vi "Drive and Climb Logging.vi"   [LabVIEW 2016]
uses:
  Robot Global Data.vi
  Drive and Climb Logging Values.vi
types:
  T1 = typedef "WPI_DriverStationRobotMode2.ctl" = enum16{"Autonomous Disabled", "Autonomous Enabled", "Teleop Disabled", "Teleop Enabled", "Disconnected", "Finish", "Test Disabled", "Test Enabled", "Emergency Stopped"}
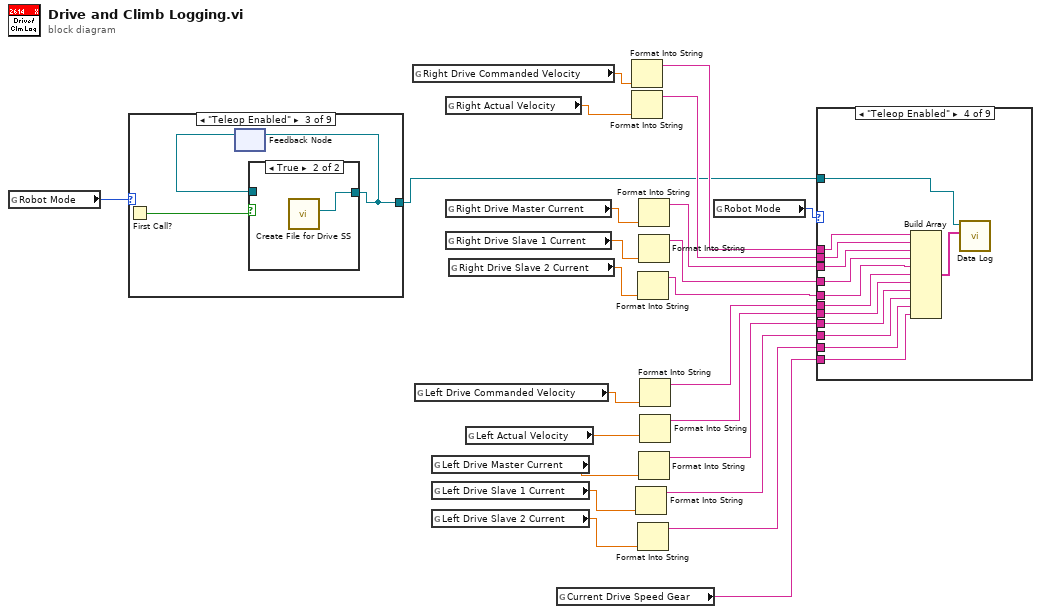
[diagram p0: block diagram]
diagram:
  n1 = global read "Robot Global Data.vi" "Robot Mode"() -> (w19:T1)
  n2 = case shown="\"Teleop Enabled\"" w19 {
    tunnel: [_ _ w25 _ _ _ _ _ _] -> w18
    frame "Autonomous Enabled" {
    }
    frame "Teleop Disabled", Default {
    }
    frame "Teleop Enabled" {
      n3 = First Call?() -> (First Call?: T/F=w27:bool)
      n4 = feedback #1() -> (w26:refnum<file>)  [unwired: 1 in]
      n5 = case shown="True" w27 {
        tunnel: [w28 w29] -> w25
        tunnel: w26 -> [w28 _]
        frame False {
        }
        frame True {
          n6 = call "Create File for Drive SS.vi"() -> ("File Reference Out"=w29:refnum<file>)  [unwired: 11 in]
        }
      }
      n7 = feedback-in #1(w25) -> ()
    }
    frame "Disconnected" {
    }
    frame "Finish" {
    }
    frame "Test Disabled" {
    }
    frame "Test Enabled" {
    }
    frame "Emergency Stopped" {
    }
    frame "Autonomous Disabled" {
    }
  }
  n8 = global read "Drive and Climb Logging Values.vi" "Right Drive Commanded Velocity"() -> (w13:dbl)
  n9 = global read "Drive and Climb Logging Values.vi" "Left Drive Commanded Velocity"() -> (w14:dbl)
  n10 = global read "Drive and Climb Logging Values.vi" "Left Drive Master Current"() -> (w12:dbl)
  n11 = global read "Drive and Climb Logging Values.vi" "Left Drive Slave 1 Current"() -> (w11:dbl)
  n12 = global read "Drive and Climb Logging Values.vi" "Left Drive Slave 2 Current"() -> (w10:dbl)
  n13 = global read "Drive and Climb Logging Values.vi" "Right Actual Velocity"() -> (w17:dbl)
  n14 = global read "Drive and Climb Logging Values.vi" "Right Drive Master Current"() -> (w6:dbl)
  n15 = global read "Drive and Climb Logging Values.vi" "Right Drive Slave 1 Current"() -> (w5:dbl)
  n16 = global read "Drive and Climb Logging Values.vi" "Right Drive Slave 2 Current"() -> (w4:dbl)
  n17 = global read "Drive and Climb Logging Values.vi" "Left Actual Velocity"() -> (w15:dbl)
  n18 = global read "Drive and Climb Logging Values.vi" "Current Drive Speed Gear"() -> (w16:string)
  n19 = Format Into String(w13) -> (resulting string=w24:string)  [unwired: 3 in, 1 out]
  n20 = Format Into String(w17) -> (resulting string=w23:string)  [unwired: 3 in, 1 out]
  n21 = Format Into String(w11) -> (resulting string=w8:string)  [unwired: 3 in, 1 out]
  n22 = Format Into String(w4) -> (resulting string=w1:string)  [unwired: 3 in, 1 out]
  n23 = Format Into String(w10) -> (resulting string=w7:string)  [unwired: 3 in, 1 out]
  n24 = Format Into String(w6) -> (resulting string=w3:string)  [unwired: 3 in, 1 out]
  n25 = Format Into String(w5) -> (resulting string=w2:string)  [unwired: 3 in, 1 out]
  n26 = Format Into String(w12) -> (resulting string=w9:string)  [unwired: 3 in, 1 out]
  n27 = Format Into String(w14) -> (resulting string=w22:string)  [unwired: 3 in, 1 out]
  n28 = Format Into String(w15) -> (resulting string=w21:string)  [unwired: 3 in, 1 out]
  n29 = global read "Robot Global Data.vi" "Robot Mode"() -> (w20:T1)
  n30 = case shown="\"Teleop Enabled\"" w20 {
    tunnel: w24 -> [_ _ _ w41 _ _ _ _ _]
    tunnel: w23 -> [_ _ _ w40 _ _ _ _ _]
    tunnel: w22 -> [_ _ _ w39 _ _ _ _ _]
    tunnel: w21 -> [_ _ _ w33 _ _ _ _ _]
    tunnel: w16 -> [_ _ _ w38 _ _ _ _ _]
    tunnel: w18 -> [_ _ _ w37 _ _ _ _ _]
    tunnel: w9 -> [_ _ _ w36 _ _ _ _ _]
    tunnel: w8 -> [_ _ _ w35 _ _ _ _ _]
    tunnel: w7 -> [_ _ _ w34 _ _ _ _ _]
    tunnel: w3 -> [_ _ _ w32 _ _ _ _ _]
    tunnel: w2 -> [_ _ _ w31 _ _ _ _ _]
    tunnel: w1 -> [_ _ _ w30 _ _ _ _ _]
    frame "Autonomous Disabled", Default {
    }
    frame "Autonomous Enabled" {
    }
    frame "Teleop Disabled" {
    }
    frame "Teleop Enabled" {
      n31 = Build Array(w41, w40, w32, w31, w30, w39, w33, w36, w35, w34, w38) -> (w42:string[])
      n32 = call "Data Log.vi"("Data In"=w42, "File Reference In"=w37) -> ()  [unwired: 9 in, 1 out]
    }
    frame "Disconnected" {
    }
    frame "Finish" {
    }
    frame "Test Disabled" {
    }
    frame "Test Enabled" {
    }
    frame "Emergency Stopped" {
    }
  }
